vi "Remove FIFO Publisher.vi"(8 "error in (no error)":errorcluster, 10 "Channel Name":string, 11 "CIFChannelMng in":refnum<class "CIFChannelMng.lvclass">) -> (0 "error out":errorcluster, 2 "FIFO Publisher":T1, 3 "CIFChannelMng out":refnum<class "CIFChannelMng.lvclass">)   [LabVIEW 2021, in "CIFChannelMng.lvclass"]
uses:
  CIFChannelMng.lvclass
  <vilib>/CIF Foundation/CIF Channels Core/CIFChannels/Typedef/Channel State.ctl
  <vilib>/CIF Foundation/CIF Channels Core/CIFChannels/CIFChannels.lvclass
  OOB/OOB_Tx/Typedef/FIFO Publisher Return.ctl
  OOB/OOB_Tx/ChnMngOOB_Tx.lvclass
  typedef/Errors Channel Manager.ctl
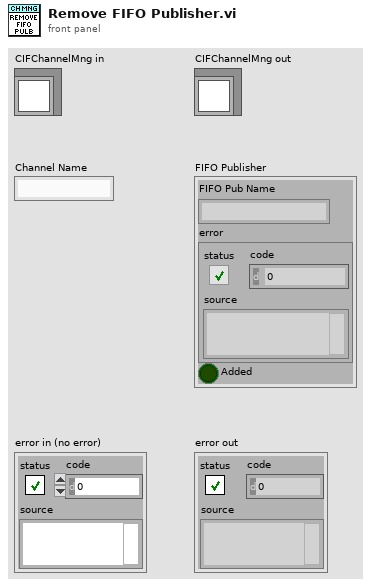
[diagram p1: front panel]
types:
  T1 = typedef "ChnMngOOB_Tx.lvclass/FIFO Publisher Return.ctl" = cluster{"FIFO Pub Name":string, "error":errorcluster, "Added":bool}
  T2 = typedef "CIFChannelMng.lvclass/Errors Channel Manager.ctl" = enum16{"gRPC Server Not Found", "Duplicate Channel", "Missing Channel", "Incorrect Type", "Flatten Error", "Unflatten Data", "Channel Length", "Plugin Connection", "gRPC Server Connection", "FIFO Unflatten", "Required Override", "Remove Not Found", "Skipped due to warning"}
  T3 = typedef "CIFChannels.lvclass/Channel State.ctl" = enum16{"Creating", "Disconnected", "Connecting", "Connected", "Destroyed"}
  T4 = typedef "CIFChannelMng.lvclass/Channel List for OOB.ctl" = cluster{"Name":string, "Direction":T5, "Type":string, "Connected?":bool, "Connected Name":string, "Custom Config Data":u8[], "Forced?":bool}
  T5 = typedef "CIFChannels.lvclass/Direction.ctl" = enum16{"Publisher", "Subscriber"}
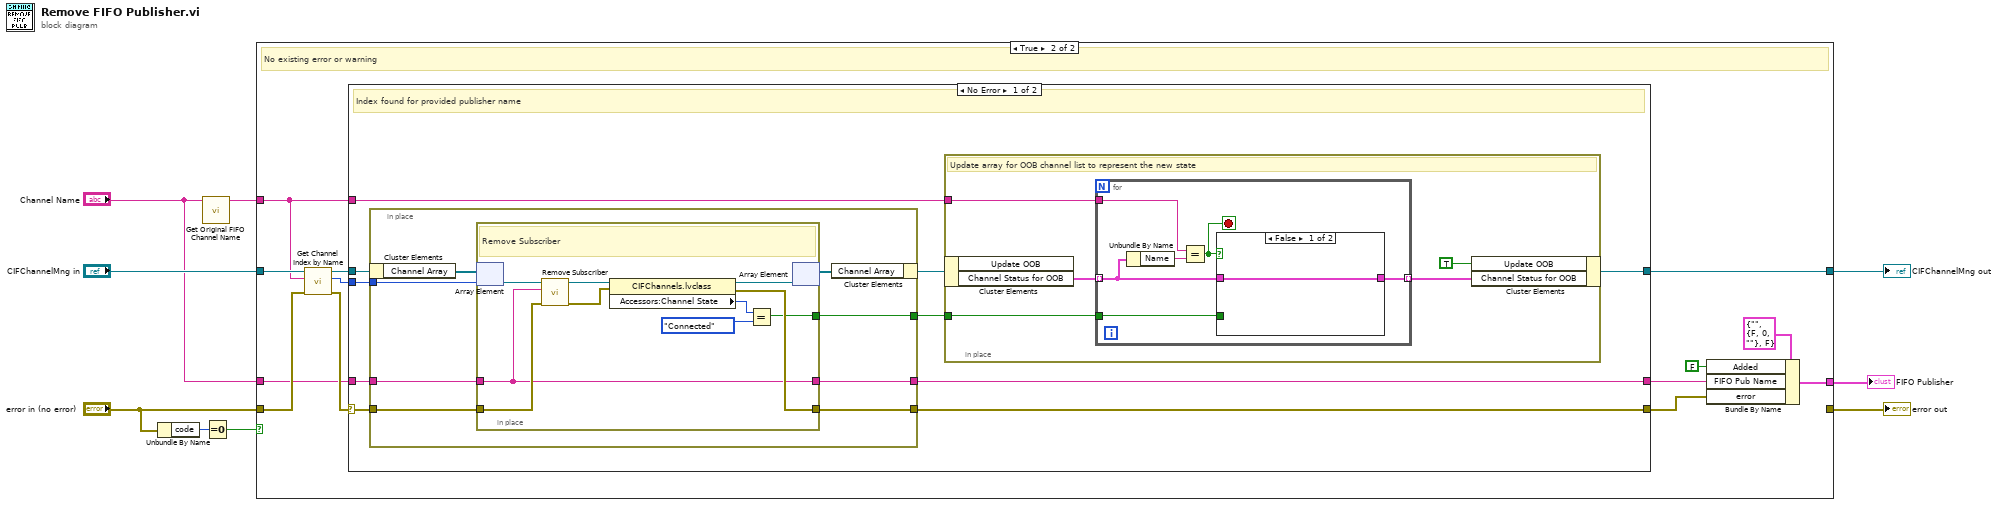
[diagram p0: block diagram]
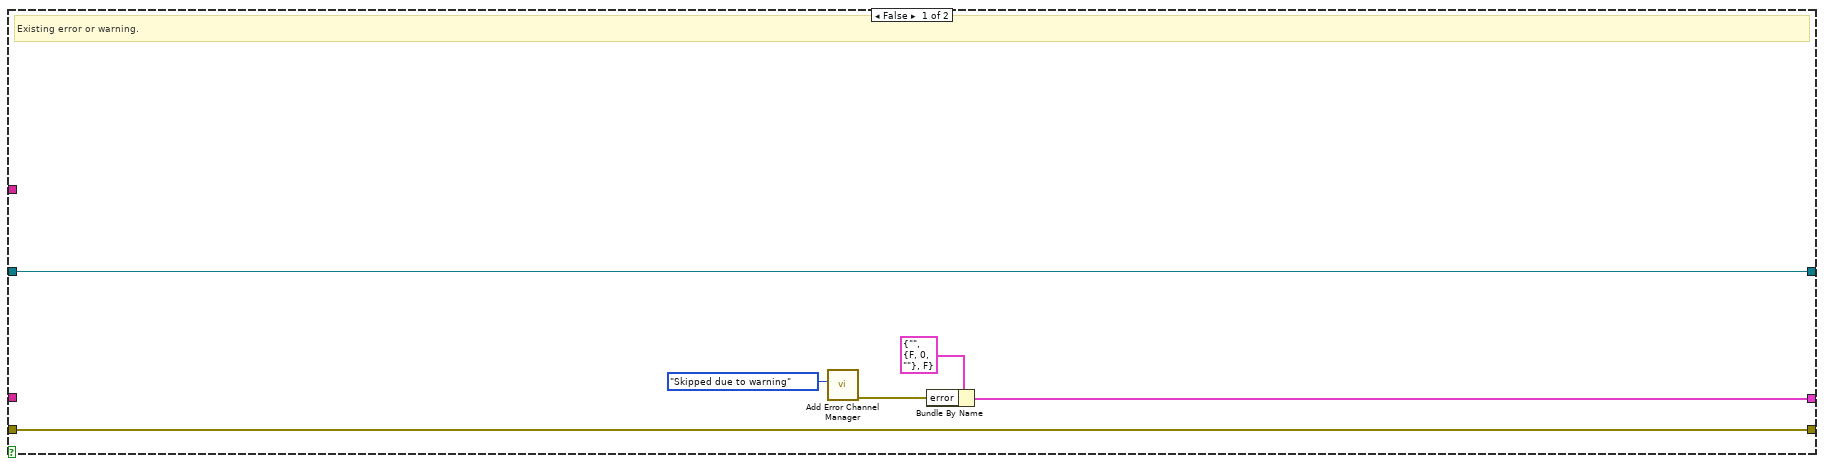
[diagram p2: hidden frame]
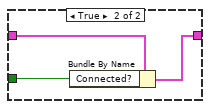
[diagram p3: hidden frame]
diagram:
  n1 = Unbundle By Name("error in (no error)") -> ("code"=w8:i32)
  n2 = call "Get Original FIFO Channel Name.vi"("Channel Name"="Channel Name") -> ("Original Channel Name"=w6:string)  [unwired: 10 in]
  n3 = Equal To 0?(x=w8) -> (x = 0?=w7:bool)
  n4 = case shown="True" w7 {
    tunnel: [w15 w24] -> w2
    tunnel: "CIFChannelMng in" -> [w15 w28]
    tunnel: w6 -> [_ w25]
    tunnel: [w14 _] -> w1
    tunnel: [w12 w19] -> w9
    tunnel: "error in (no error)" -> [w14 w18]
    tunnel: "Channel Name" -> [_ w16]
    frame False {
      # "Existing error or warning."
      n5 = call "Add Error Channel Manager.vi"("Error"=Errors_Channel_Manager."Skipped due to warning") -> ("error out"=w11:errorcluster)  [unwired: 10 in]
      n6 = Bundle By Name(cluster=T1 {"FIFO Pub Name"="", "error"={"status"=FALSE, "code"=0, "source"=""}, "Added"=FALSE} ("New FIFO Publisher"), "error"=w11) -> (w12:T1)
    }
    frame True {
      # "No existing error or warning"
      n7 = call "Get Channel Index by Name.vi"("error in (no error)"=w18, "Channel Name"=w25, "CIFChannelMng in"=w28) -> ("error out"=w23:errorcluster, "Channel Index"=w26:i32, "CIFChannelMng out"=w27:refnum<class "CIFChannelMng.lvclass">)  [unwired: 6 in]
      n8 = case shown="No Error" w23 {
        selector: w23 -> [w31 w73]
        tunnel: w27 -> [w38 w72]
        tunnel: w26 -> [w37 _]
        tunnel: w25 -> [w35 _]
        tunnel: [w34 w72] -> w24
        tunnel: [w33 w73] -> w20
        tunnel: w16 -> [w32 _]
        tunnel: [w29 _] -> w21
        frame No Error {
          # "Index found for provided publisher name"
          n9 = in-place {
            in-place-border: w37 -> [w60]
            in-place-border: w31 -> [w59]
            in-place-border: [w57] -> w33
            in-place-border: w32 -> [w56]
            in-place-border: [w55] -> w30
            in-place-border: [w54] -> w29
            n10 = in-place-cluster #1(w38) -> ("Channel Array"=w61:refnum<class "CIFChannels.lvclass">[])
            n11 = in-place {
              in-place-border: w59 -> [w64]
              in-place-border: [w70] -> w57
              in-place-border: w56 -> [w62]
              in-place-border: [w67] -> w55
              in-place-border: [w62] -> w54
              # "Remove Subscriber"
              n12 = in-place-array #2(w61, w60) -> (w66:refnum<class "CIFChannels.lvclass">)
              n13 = call-dynamic "Remove Subscriber.vi"("error in (no error)"=w64, "Publisher to Remove"=w62, "CIFChannels in"=w66) -> ("error out"=w63:errorcluster, "CIFChannels out"=w65:refnum<class "CIFChannels.lvclass">)  [unwired: 7 in]
              n14 = property class="CIFChannels.lvclass"(reference=w65, error in=w63) -> (reference out=w71:refnum<class "CIFChannels.lvclass">, error out=w70:errorcluster, "Accessors:Channel State"=w68:T3)
              n15 = Equal?(x=w68, y=Channel_State."Connected" ("Channel State")) -> (x = y?=w67:bool)
              n16 = in-place-array #2(w71) -> (w58:refnum<class "CIFChannels.lvclass">[])  [unwired: 1 out]
            }
            n17 = in-place-cluster #1("Channel Array"=w58) -> (w36:refnum<class "CIFChannelMng.lvclass">)
          }
          n18 = in-place {
            in-place-border: w35 -> [w40]
            in-place-border: w30 -> [w39]
            # "Update array for OOB channel list to represent the new state"
            n19 = in-place-cluster #3(w36) -> ("Channel Status for OOB"=w43:T4[])  [unwired: 1 out]
            n20 = for {
              tunnel: w43 -> [w48] mode=indexing
              tunnel: [w47] -> w42 mode=indexing
              tunnel: w40 -> [w46]
              tunnel: w39 -> [w44]
              stop <- w45 stop-if-true
              n21 = Unbundle By Name(w48) -> ("Name"=w49:string)
              n22 = Equal?(x=w46, y=w49) -> (x = y?=w45:bool)
              n23 = case shown="False" w45 {
                tunnel: w48 -> [w50 w53]
                tunnel: [w50 w52] -> w47
                tunnel: w44 -> [_ w51]
                frame False {
                }
                frame True {
                  n24 = Bundle By Name(cluster=w53, "Connected?"=w51) -> (w52:T4)
                }
              }
            }
            n25 = in-place-cluster #3("Update OOB"=TRUE, "Channel Status for OOB"=w42) -> (w34:refnum<class "CIFChannelMng.lvclass">)
          }
        }
        frame Error {
          # "Index by name created error"
        }
      }
      n26 = Bundle By Name(cluster=T1 {"FIFO Pub Name"="", "error"={"status"=FALSE, "code"=0, "source"=""}, "Added"=FALSE} ("New FIFO Publisher"), "Added"=FALSE, "FIFO Pub Name"=w21, "error"=w20) -> (w19:T1)
    }
  }
  "error out" <- w1
  "CIFChannelMng out" <- w2
  "FIFO Publisher" <- w9
